vi "dF(e)_dt.vi"(7 "Function":enum16{"Linear", "Sigmoid", "Tangent hyp."}(ring)=enum."Sigmoid", 11 "yout":sgl) -> (3 "New Weight":sgl)   [LabVIEW 2012]
panel:
  # "Chuck Streb Dec2007"
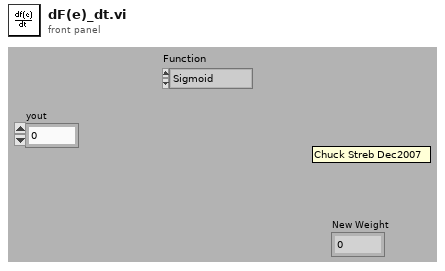
[diagram p1: front panel]
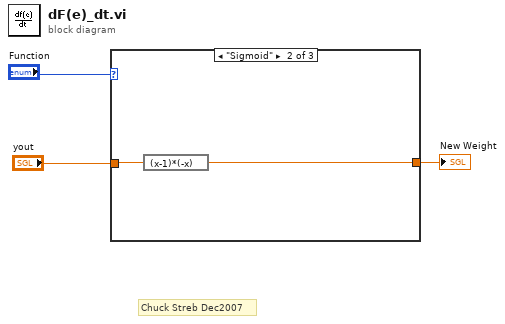
[diagram p0: block diagram]
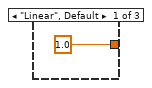
[diagram p2: hidden frame]
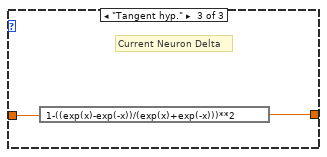
[diagram p3: hidden frame]
diagram:
  # "Chuck Streb Dec2007"
  n1 = case shown="\"Sigmoid\"" "Function" {
    tunnel: "yout" -> [_ w6 w8]
    tunnel: [sgl 1.0 w5 w7] -> w1
    frame "Linear", Default {
    }
    frame "Sigmoid" {
      n2 = expression code="(x-1)*(-x)"(w6) -> (w5:sgl)
    }
    frame "Tangent hyp." {
      # "Current Neuron Delta"
      n3 = expression code="1-((exp(x)-exp(-x))/(exp(x)+exp(-x)))**2"(w8) -> (w7:sgl)
    }
  }
  "New Weight" <- w1
